vi "Euler.vi"(9 "dt":dbl, 11 "x":dbl) -> (3 "x'":dbl)   [LabVIEW 2012]
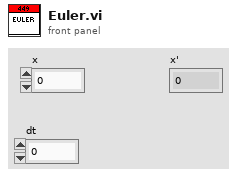
[diagram p1: front panel]
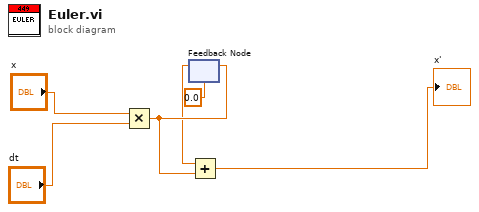
[diagram p0: block diagram]
diagram:
  n1 = Multiply(x="x", y="dt") -> (x*y=w3:dbl)
  n2 = feedback-in #1(w3) -> ()
  n3 = feedback #1(0.0) -> (w2:dbl)
  n4 = Add(x=w2, y=w3) -> (x+y=→"x'":dbl)
